vi "ET3500 - Read Registers.vi"(4 "Simulate":bool, 5 "ET3500 Segment Enum":T1 items=["Segment.Type", "Segment.Holdback", "", "", "Segment.Duration", "Segment.RampRate", "Segment.TargetSP", "Segment.EndAction", "", "", "", "", "", "", "", "", "Segment.GsoakType", "Segment.GsoakVal"], 6 "Option":cluster{"Init":bool, "Close":bool}, 7 "ET3500 Programmer Enum":T2 items=["Comms.ProgramNumber", "", "Program.RampUnits", "Program.DwellUnits", "", "", "", "", "", "Programmer.CurProg", "Programmer.CurSeg", "Programmer.ProgStatus", "", "", "", "", "", "Programmer.ProgTimeLeft", "Programmer.PVIn", "Programmer.SPIn", "", "Programmer.SegTimeLeft"], 8 "error in (no error)":errorcluster, 9 "Num Of Reg (1)":u16=1, 10 "ET3500 Enum":T3, 11 "VISA resource name":refnum<visa-resource-name>="COM3") -> (0 "error out":errorcluster, 1 "Data Array":i16[](array[numeric]), 2 "Data":i16, 3 "VISA resource name out":refnum<visa-resource-name>)   [LabVIEW 2013]
uses:
  Controls/ET3500 Enum.ctl
  Controls/ET3500 Programmer Enum.ctl
  Controls/ET3500 Segment Enum.ctl
  <instrlib>/Eurotherm 35xx Series/Eurotherm 35xx Series.lvlib
panel:
  # "Segment1\n5376\n(0-23)"
  # "Programmer1\n5184\n(0-45)"
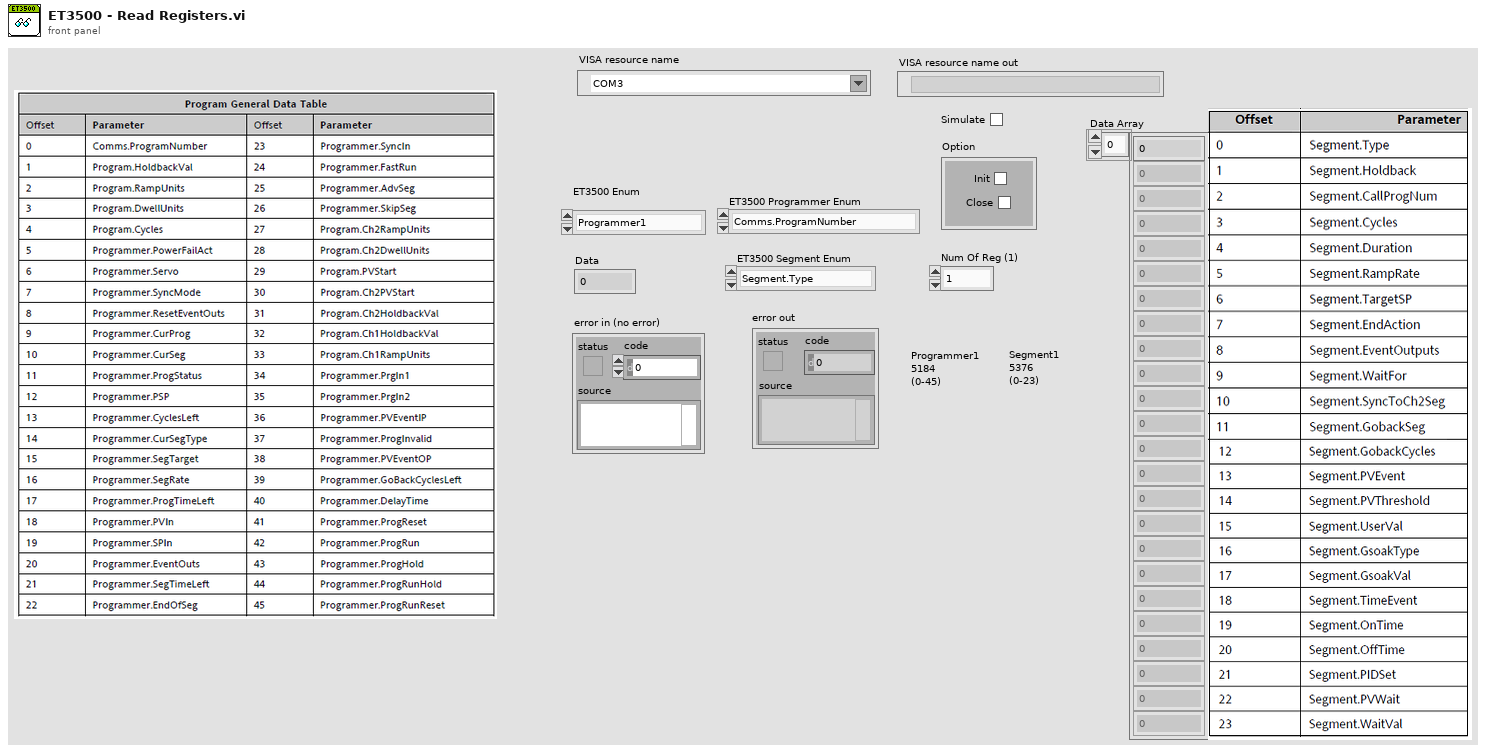
[diagram p1: front panel]
types:
  T1 = typedef "ET3500 Segment Enum.ctl" = u16
  T2 = typedef "ET3500 Programmer Enum.ctl" = u16
  T3 = typedef "ET3500 Enum.ctl" = enum16{"Programmer1", "Segment1", "Segment2", "Segment3", "Segment4", "Segment5", "Segment6", "Segment7", "Segment8", "Segment9", "Segment10", "Segment11", "Segment12", "Segment13", "Segment14", "Segment15", "Segment16"}
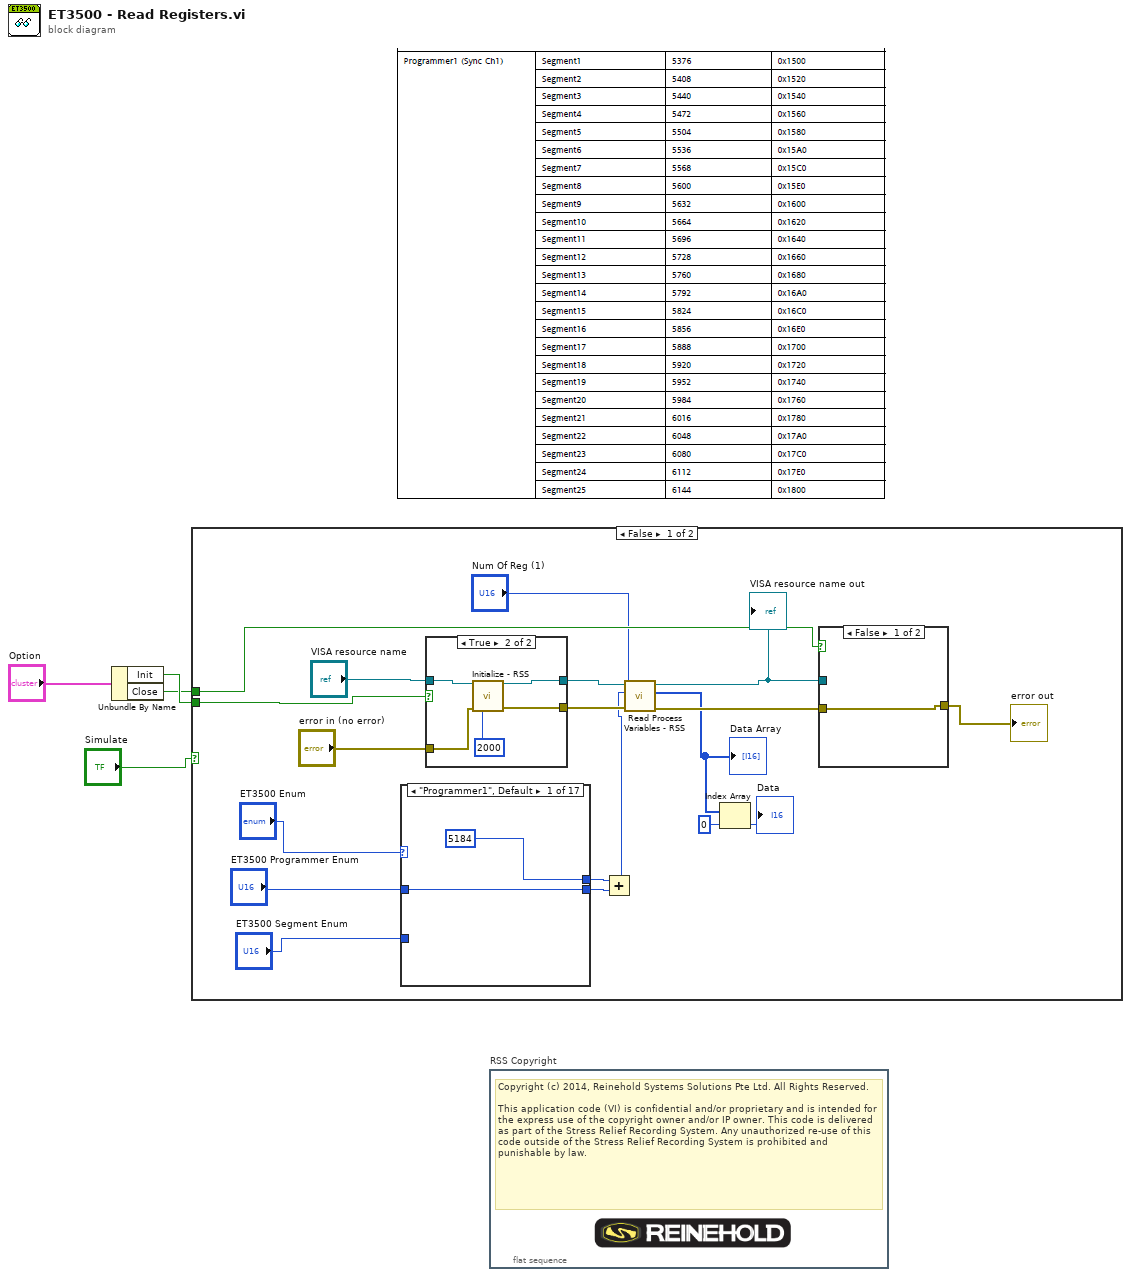
[diagram p0: block diagram]
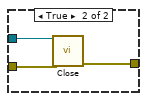
[diagram p2: hidden frame]
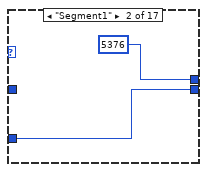
[diagram p4: hidden frame]
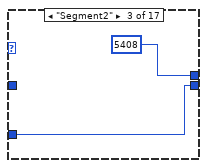
[diagram p5: hidden frame]
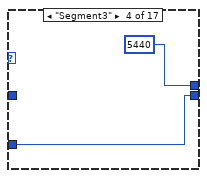
[diagram p6: hidden frame]
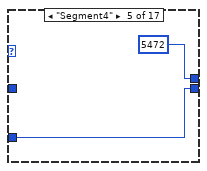
[diagram p7: hidden frame]
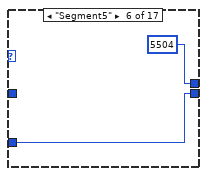
[diagram p8: hidden frame]
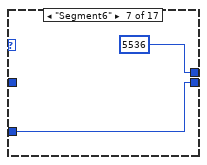
[diagram p9: hidden frame]
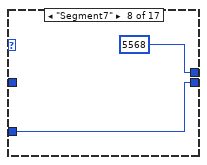
[diagram p10: hidden frame]
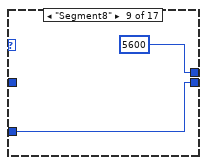
[diagram p11: hidden frame]
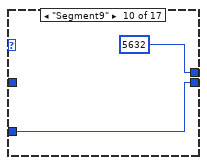
[diagram p12: hidden frame]
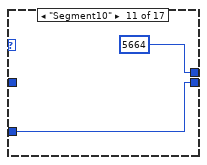
[diagram p13: hidden frame]
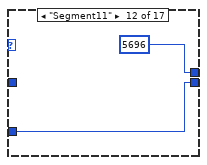
[diagram p14: hidden frame]
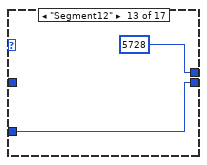
[diagram p15: hidden frame]
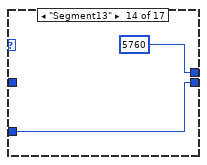
[diagram p16: hidden frame]
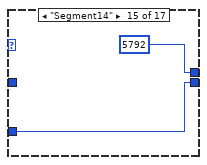
[diagram p17: hidden frame]
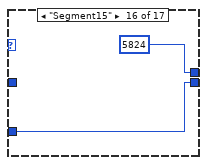
[diagram p18: hidden frame]
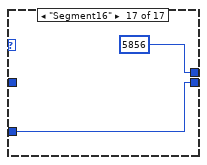
[diagram p19: hidden frame]
diagram:
  n1 = Unbundle By Name("Option") -> ("Init"=w3:bool, "Close"=w2:bool)
  n2 = case shown="False" "Simulate" {
    tunnel: w3 -> [w8 _]
    tunnel: w2 -> [w7 _]
    frame False {
      n3 = case shown="\"Programmer1\", Default" "ET3500 Enum" {
        tunnel: "ET3500 Programmer Enum" -> [w35 _ _ _ _ _ _ _ _ _ _ _ _ _ _ _ _]
        tunnel: [u16 5184 ("Register Address (0)") u16 5376 ("Register Address (0)") u16 5408 ("Register Address (0)") u16 5440 ("Register Address (0)") u16 5472 ("Register Address (0)") u16 5504 ("Register Address (0)") u16 5536 ("Register Address (0)") u16 5568 ("Register Address (0)") u16 5600 ("Register Address (0)") u16 5632 ("Register Address (0)") u16 5664 ("Register Address (0)") u16 5696 ("Register Address (0)") u16 5728 ("Register Address (0)") u16 5760 ("Register Address (0)") u16 5792 ("Register Address (0)") u16 5824 ("Register Address (0)") u16 5856 ("Register Address (0)")] -> w17
        tunnel: [w35 w37 w39 w41 w44 w45 w48 w50 w52 w54 w56 w58 w60 w62 w64 w66 w68] -> w16
        tunnel: "ET3500 Segment Enum" -> [_ w37 w39 w41 w44 w45 w48 w50 w52 w54 w56 w58 w60 w62 w64 w66 w68]
        frame "Programmer1", Default {
        }
        frame "Segment1" {
        }
        frame "Segment2" {
        }
        frame "Segment3" {
        }
        frame "Segment4" {
        }
        frame "Segment5" {
        }
        frame "Segment6" {
        }
        frame "Segment7" {
        }
        frame "Segment8" {
        }
        frame "Segment9" {
        }
        frame "Segment10" {
        }
        frame "Segment11" {
        }
        frame "Segment12" {
        }
        frame "Segment13" {
        }
        frame "Segment14" {
        }
        frame "Segment15" {
        }
        frame "Segment16" {
        }
      }
      n4 = case shown="True" w8 {
        tunnel: [w28 w34] -> w23
        tunnel: [w29 w33] -> w22
        tunnel: "VISA resource name" -> [w29 w32]
        tunnel: "error in (no error)" -> [w28 w31]
        frame False {
        }
        frame True {
          n5 = call <instrlib>:"Initialize - RSS.vi"("VISA resource name"=w32, "error in (no error)"=w31, "General Settings:Timeout Value"=u32 2000) -> ("VISA resource name out"=w33:refnum<visa-resource-name>, "error out"=w34:errorcluster)  [unwired: 11 in]
        }
      }
      n6 = Add(x=w17, y=w16) -> (x+y=w14:T1)
      n7 = call "Read Process Variables - RSS.vi"("error in (no error)"=w23, "Num Of Reg (1)"="Num Of Reg (1)", "Register Address (0)"=w14, "VISA resource name"=w22) -> ("error out"=w20:errorcluster, "Data"=w13:i16[], "VISA resource name out"=w21:refnum<visa-resource-name>)  [unwired: 5 in]
      "Data Array" <- w13
      "VISA resource name out" <- w21
      n8 = Index Array(array=w13, index=0) -> (element=→"Data":i16)
      n9 = case shown="False" w7 {
        tunnel: w21 -> [_ w27]
        tunnel: w20 -> [w24 w26]
        tunnel: [w24 w25] -> w10
        frame False {
        }
        frame True {
          n10 = call <instrlib>:"Close.vi"("VISA resource name"=w27, "error in (no error)"=w26) -> ("error out"=w25:errorcluster)  [unwired: 13 in]
        }
      }
      "error out" <- w10
    }
    frame True {
    }
  }
  n11 = flat-sequence "RSS Copyright" {
    frame #0 {
      # "Copyright (c) 2014, Reinehold Systems Solutions Pte Ltd. All Rights Reserved.\n\nThis application code (VI) is confidential and/or proprietary and is intended for the express use of the copyright owner and/or IP owner. This code is delivered as part of the Stress Relief Recording System. Any unauthorized re-use of this code outside of the Stress Relief Recording System is prohibited and punishable by law."
    }
  }
